vi "Pre Launch Init.vi"(11 "Door Hardware in":refnum<class "Door Hardware.lvclass">) -> (0 "error out":errorcluster, 3 "Door Hardware out":refnum<class "Door Hardware.lvclass">)   [LabVIEW 2020, in "Door Hardware.lvlib" / "Door Hardware.lvclass"]
doc: "(<B>Filename</B>: Actor Framework.lvlib:Actor.lvclass:Pre Launch Init.vi)\n\nDefines behavior that occurs after the Launch Nested Actor method is invoked but before the actor's Actor Core method begins running.\n\nBy default, this method does nothing. A descendant class may override it to define behavior."
uses:
  Door Hardware.lvclass
  C:/Program Files/National Instruments/LabVIEW 2020/vi.lib/ActorFramework/Actor/Actor.lvclass
  <vilib>/ActorFramework/Actor/Actor.lvclass/Actor.ctl
  <vilib>/ActorFramework/Message Enqueuer/Message Enqueuer.lvclass/Message Enqueuer.ctl
  Simulated Actuator/Simulated Actuator.lvclass
  C:/Users/Thomas.McQuillan/Desktop/Elevator Door Control/Door Actuator/Door Actuator.lvclass
  Simulated Interlocks/Simulated Interlocks.lvclass
  C:/Users/Thomas.McQuillan/Desktop/Elevator Door Control/Door Interlocks/Door Interlocks.lvclass
  Door Hardware Messages/Read Interlock Status Msg/Read Interlock Status Msg.lvclass
  C:/Program Files/National Instruments/LabVIEW 2020/vi.lib/ActorFramework/Message/Message.lvclass
  Door Hardware.lvclass/Door Hardware.ctl
  <vilib>/ActorFramework/Time-Delayed Send Message/Time-Delay Override Options.ctl
  <vilib>/ActorFramework/Message Enqueuer/Init from Existing Queue.vi
  <vilib>/ActorFramework/Message Enqueuer/Message Enqueuer.lvclass
  Application/Application/Application.lvclass
  <vilib>/ActorFramework/Actor/Actor.lvclass
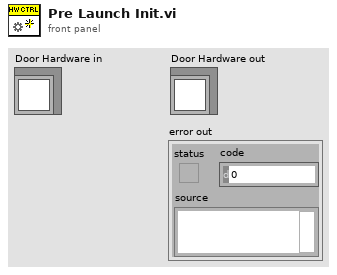
[diagram p1: front panel]
types:
  T1 = typedef "Door Interlocks.lvclass/Interlock Values.ctl" = cluster{"Door Open":bool, "Door Closed":bool, "Mode of Operation":T2}
  T2 = typedef "Door Interlocks.lvclass/Mode of Operation.ctl" = enum16{"Standard", "Interlock Override"}
  T3 = typedef "Time-Delay Override Options.ctl" = enum16{"Send next copy now", "Skip next scheduled copy", "Send next copy now and stop all further copies", "Stop all further copies"}
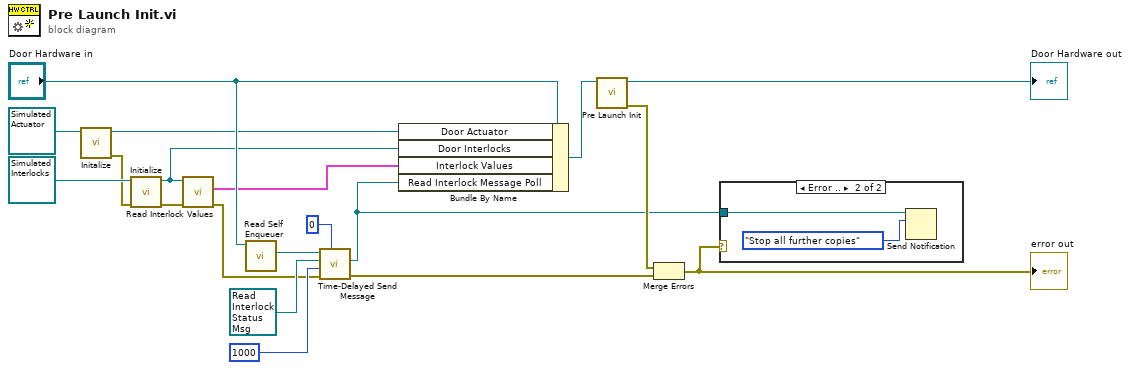
[diagram p0: block diagram]
diagram:
  n1 = call-dynamic "Initalize.vi"("Simulated Actuator in"=refnum<class "Simulated Actuator.lvclass"> refnum ("Simulated Actuator.lvclass")) -> ("error out"=w5:errorcluster, "Simulated Actuator out"=w6:refnum<class "Simulated Actuator.lvclass">)  [unwired: 9 in]
  n2 = call-dynamic "Initialize.vi"("error in (no error)"=w5, "Simulated Interlocks in"=refnum<class "Simulated Interlocks.lvclass"> refnum ("Simulated Interlocks.lvclass")) -> ("error out"=w2:errorcluster, "Simulated Interlocks out"=w3:refnum<class "Simulated Interlocks.lvclass">)  [unwired: 8 in]
  n3 = call-dynamic "Read Interlock Values.vi"("error in (no error)"=w2, "Simulated Interlocks in"=w3) -> ("error out"=w1:errorcluster, "Interlock Values"=w4:T1)  [unwired: 8 in]
  n4 = call <vilib>:"Read Self Enqueuer.vi"("Actor"="Door Hardware in") -> ("Self Enqueuer"=w15:refnum<class "Message Enqueuer.lvclass">)  [unwired: 10 in]
  n5 = call <vilib>:"Time-Delayed Send Message.vi"("# Copies (0 = infinite repeat)"=u32 0, "error in (no error)"=w1, "Milliseconds To Wait"=1000, "Message"=refnum<class "Read Interlock Status Msg.lvclass"> refnum ("Door Hardware.lvlib:Read Interlock Status Msg.lvclass"), "Message Enqueuer"=w15) -> ("error out"=w12:errorcluster, "Delivery Notifier"=w9:refnum<notifier>)  [unwired: 5 in]
  n6 = Bundle By Name(cluster="Door Hardware in", "Door Actuator"=w6, "Door Interlocks"=w3, "Interlock Values"=w4, "Read Interlock Message Poll"=w9) -> (w18:refnum<class "Door Hardware.lvclass">)
  n7 = call-parent "Pre Launch Init.vi"("Actor in"=w18) -> ("error out"=w13:errorcluster, "Actor out"=→"Door Hardware out":refnum<class "Door Hardware.lvclass">)  [unwired: 9 in]
  n8 = Merge Errors(w13, w12) -> (w10:errorcluster)
  "error out" <- w10
  n9 = case shown="Error .." w10 {
    tunnel: w9 -> [_ w21]
    frame No Error {
    }
    frame Error {
      n10 = Send Notification(notification=Time-Delay_Override_Options."Stop all further copies", notifier=w21) -> ()  [unwired: 1 in, 2 out]
    }
  }
